vi "Test inner FIFO success.vi"() -> ()   [LabVIEW 2015]
uses:
  <vilib>/visionFPGA/Controls/IMAQ FPGA Image Size.ctl
  <vilib>/Platform/TimedLoop/XDataNode/timing_clust.ctl
  <vilib>/Platform/TimedLoop/XDataNode/nitl_modes.ctl
  <vilib>/Platform/TimedLoop/XDataNode/wakeup.ctl
  <vilib>/rvi/Emulation/niFpgaSctlEmulationGetInTimedLoop.vi
  <vilib>/rvi/Emulation/niFpgaEmulationReportErrorSimple.vi
  <vilib>/rvi/Emulation/niFpgaGetClockAttributes.vi
  <vilib>/rvi/Emulation/niFpgaCriticalErrorInLSC.vi
  <vilib>/rvi/DataTransferAndStorage/Container/Common/niFpgaContainerGetUniqueNameForEmu.vi
  <vilib>/rvi/DataTransferAndStorage/Container/Common/niFpgaContainerSetEmuInfo.vi
  <vilib>/rvi/eio/common/nirviEmuReportErrorAndStop.vi
  <vilib>/visionFPGA/Basics/FIFO to Pixel Bus/IMAQ FPGA FIFO to Pixel Bus RGB32x1.vi
  <vilib>/visionFPGA/Basics/Pixel Bus to FIFO/IMAQ FPGA Pixel Bus to FIFO U8x1.vi
  <vilib>/rvi/DataTransferAndStorage/Container/Common/niFpgaContainerExecOnDevCompGetState.vi
  <vilib>/rvi/Emulation/niFpgaEmulationIsFPGAContextNoSignature.vi
  <vilib>/rvi/errors/niFpgaSetErrorForExecOnDevCompSimple.vi
  <vilib>/rvi/FIFO/Fifo_Resource/nirvififoEmulationSetSize.vi
  <vilib>/rvi/FIFO/Fifo_Resource/nirviFifoEmulationQueueMgr.vi
  <instcachedir>/0/nirviFifoEmulationQueueMgr_E5CAEC123FF24DC58D834DCA3CDAA9B5.lvgen/nirviFifoEmulationQueueMgr_E5CAEC123FF24DC58D834DCA3CDAA9B5_001.vi
  <vilib>/rvi/FIFO/Fifo_Resource/nirvififoEmulationDetermineInputValidOut.vi
  <vilib>/rvi/FIFO/Fifo_Resource/nirvififoEmulationCreateLock.vi
  <vilib>/rvi/Emulation/niFpgaProcessEmulError.vi
  <vilib>/rvi/FIFO/Fifo_Resource/nirvififoEmulationObtainLock.vi
  <vilib>/rvi/FIFO/Fifo_Resource/nirvififoEmulationReleaseLock.vi
  <vilib>/rvi/occurrence/nirviWaitOnOccurrenceBase.vi
  <vilib>/rvi/errors/nirviReportUnexpectedCaseInternalError.vi
  <vilib>/rvi/errors/nirviReportUnexpectedCaseInternalError (U32).vi
  <vilib>/Utility/error.llb/Clear Errors.vi
  <vilib>/rvi/interface/RandomDataEmulation/niFpgaRandomDataHandleErrors.vi
  <vilib>/Platform/TimedLoop/XDataNode/XDataNode.xnode
  <vilib>/rvi/LocalResourceManager/LocalResourceManager.xnode
  <vilib>/rvi/DataTransferAndStorage/Container/XNode/niFpgaContainer.xnode
  <vilib>/rvi/FIFO/Fifo_Resource/niFpgaFifoEmulationRefIn.vi
  <vilib>/visionFPGA/NI_VDM_FPGA_Basics.lvlib
  <vilib>/Platform/TimedLoop/XDataNode/XDNodeRunTimeDep.lvlib
panel:
  out "appended array 2":u8[](array[numeric])
  out "appended array":i16[](array[numeric])
  out "Element":i16
  out "Output Valid":bool
  out "Pixel Data":u8
  out "Line count":i16
  in  "Image Size":T1={"Width"=640, "Height"=480}
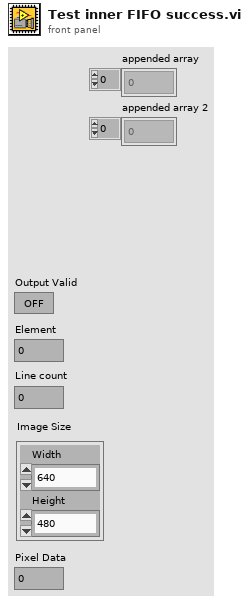
[diagram p1: front panel]
types:
  T1 = typedef "IMAQ FPGA Image Size.ctl" = cluster{"Width":u32, "Height":u32}
  T2 = typedef "XDNodeRunTimeDep.lvlib/timing_clust.ctl" = cluster{"Expected End [f-1]":u64, "Actual End [f-1]":u64, "Finished Late? [f-1]":bool, "Expected End [i-1]":u64, "Actual End [i-1]":u64, "Finished Late? [i-1]":bool, "Expected Start [i]":u64, "Actual Start [i]":u64, "Expected Start [f]":u64, "Actual Start [f]":u64, "Source Name":string, "Structure Name":string, "Period":i64, "Deadline":i64, "Offset":i64, "Start":i64, "Priority":i32, "Timeout":i32, "Mode":T3, "Wakeup Reason":T4, "Error":errorcluster, "Source Type":string, "Secondary Source Type":string, "Global End Time":u64, "Global Start Time":u64, "Frame Duration":u64, "Iteration Duration":u64, "Assigned CPU":i32, "I/O Scan Engine Mode":u32}
  T3 = typedef "XDNodeRunTimeDep.lvlib/nitl_modes.ctl" = enum32{"No Change", "Process missed periods, maintain original phase", "Discard missed periods, maintain original phase", "Process missed periods, ignore original phase", "Discard missed periods, ignore original phase"}
  T4 = typedef "XDNodeRunTimeDep.lvlib/wakeup.ctl" = enum32{"Normal", "Aborted", "Asynchronous wakeup", "Timing source error", "Timed loop error", "Timeout"}
  T5 = typedef "IMAQ FPGA Pixel Bus RGB32x1.ctl" = cluster{"Pixel Data":cluster{"A":u8, "R/H":u8, "G/S":u8, "B/L":u8}, "DV":bool, "EOL":bool, "EOI":bool, "Data Type":enum16{"RGB32 x 1"}}
  T6 = typedef "IMAQ FPGA Pixel Bus u8x1.ctl" = cluster{"Pixel Data":u8, "DV":bool, "EOL":bool, "EOI":bool, "Data Type":enum16{"U8 x 1"}}
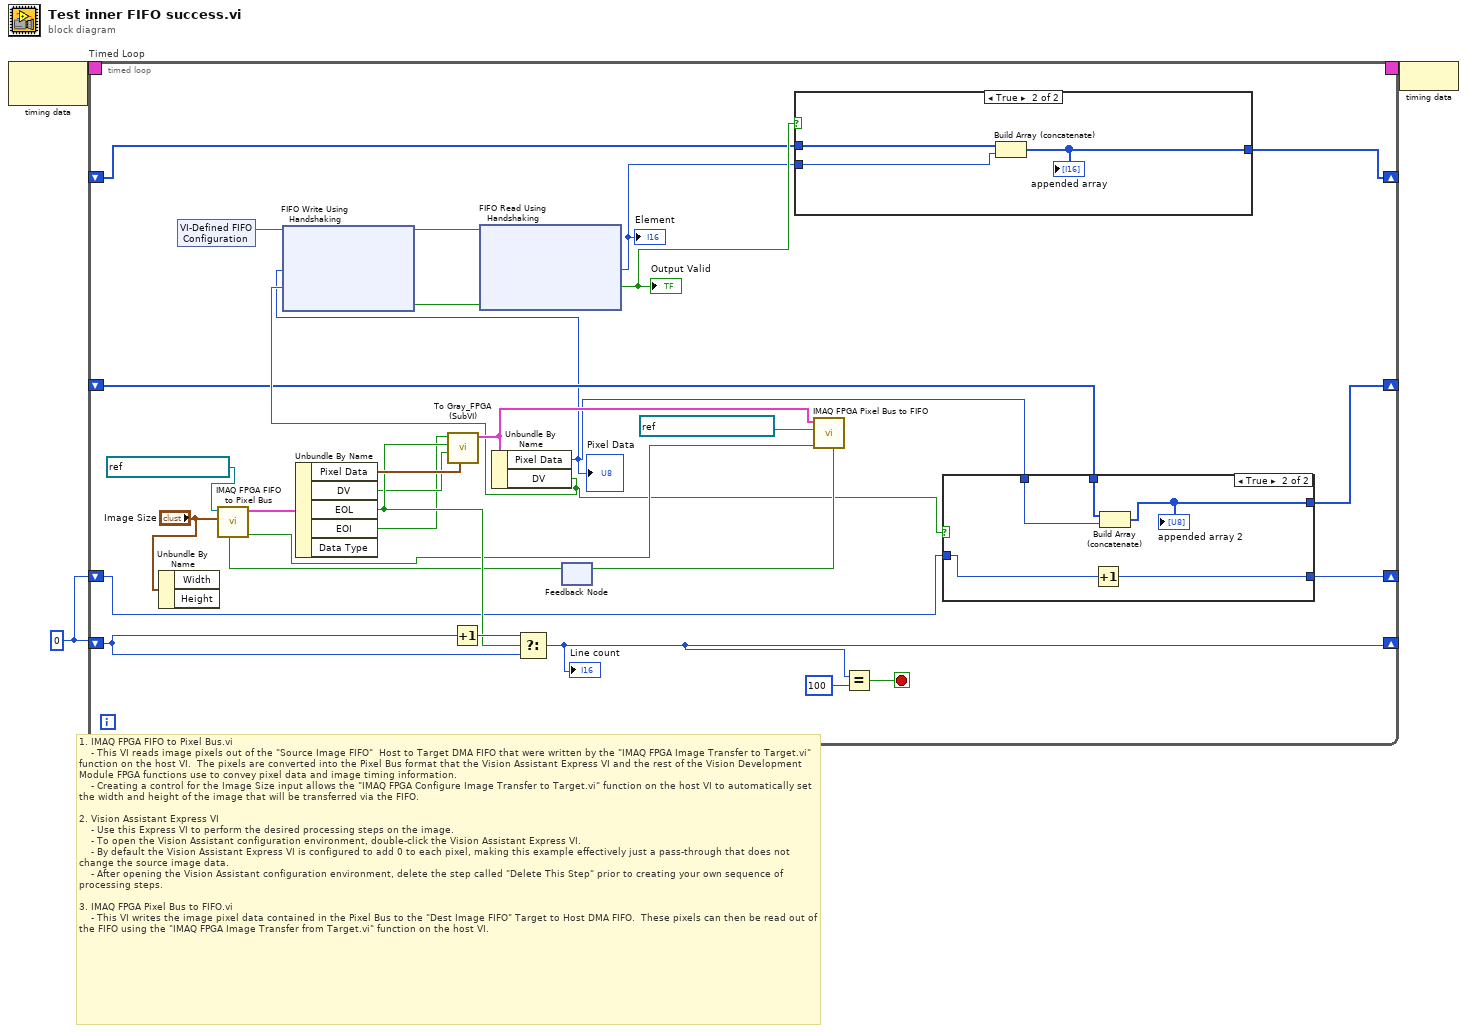
[diagram p0: block diagram]
diagram:
  w1 = i16 0
  # "1. IMAQ FPGA FIFO to Pixel Bus.vi\n    - This VI reads image pixels out of the \"Source Image FIFO\"  Host to Target DMA FIFO that were written by the \"IMAQ FPGA Image Transfer to Target.vi\" function on the host VI.  The pixels are converted into the Pixel Bus format that the Vision Assistant Express VI and the rest of the Vision Development Module FPGA functions use to convey pixel data and image timing information.\n    - Creating a control for the Image Size input allows the \"IMAQ FPGA Configure Image Transfer to Target.vi\" function on the host VI to automatically set the width and height of the image that will be transferred via the FIFO.\n\n2. Vision Assistant Express VI\n    - Use this Express VI to perform the desired processing steps on the image.\n    - To open the Vision Assistant configuration environment, double-click the Vision Assistant Express VI.\n    - By default the Vision Assistant Express VI is configured to add 0 to each pixel, making this example effectively just a pass-through that does not change the source image data.\n    - After opening the Vision Assistant configuration environment, delete the step called \"Delete This Step\" prior to creating your own sequence of processing steps.\n\n3. IMAQ FPGA Pixel Bus to FIFO.vi\n    - This VI writes the image pixel data contained in the Pixel Bus to the \"Dest Image FIFO\" Target to Host DMA FIFO.  These pixels can then be read out of the FIFO using the \"IMAQ FPGA Image Transfer from Target.vi\" function on the host VI."
  n1 = node-c288() -> (w3:T2)  [unwired: 1 in]
  n2 = timed-loop "Timed Loop" {
    timing: w3 -> [_]
    timing-out: [_] -> w2
    shift-right: [w12] -> _
    shift-left: w1 -> [w28]
    shift-right: [w15] -> _
    shift-left: w1 -> [w16]
    shift-right: [w8] -> _
    shift-left: _ -> [w7]
    shift-right: [w4] -> _
    shift-left: _ -> [w6]
    stop <- w13 stop-if-true
    n3 = Unbundle By Name("Image Size") -> ()  [unwired: 2 out]
    n4 = xnode "VI-Defined FIFO Configuration"() -> ("FIFO Out"=w20:refnum<k21>)
    n5 = Increment(x=w28) -> (x+1=w29:i16)
    n6 = feedback #1() -> (w21:bool)  [unwired: 1 in]
    n7 = call-poly <vilib>:"IMAQ FPGA FIFO to Pixel Bus.vi"("Ready For Output"=w21, "Image Size"="Image Size", "Source Image FIFO"=refnum<k21> "32it Source FIFO") -> ("Output Valid"=w23:bool, "Pixel Bus Out"=w31:T5)  [unwired: 6 in, 1 out]
    n8 = Unbundle By Name(w31) -> ("Pixel Data"=w27:cluster{"A":u8, "R/H":u8, "G/S":u8, "B/L":u8}, "DV"=w25:bool, "EOL"=w26:bool, "EOI"=w17:bool)  [unwired: 1 out]
    n9 = call "To Gray_FPGA (SubVI).vi"("Pixel Data"=w27, "DV"=w25, "EOL"=w26, "EOI"=w17) -> ("Pixel Bus In"=w24:T6)  [unwired: 7 in]
    n10 = Unbundle By Name(w24) -> ("Pixel Data"=w5:u8, "DV"=w14:bool)
    "Pixel Data" <- w5
    n11 = xnode ("FIFO Write Using Handshaking")("Element"=w5, "Input Valid"=w14, "FIFO In"=w20) -> ("Ready for Input"=w18:bool, "FIFO Out"=w19:refnum<k21>)
    n12 = xnode ("FIFO Read Using Handshaking")("Ready for Output"=w18, "FIFO In"=w19) -> ("Element"=w9:i16, "Output Valid"=w10:bool)  [unwired: 1 out]
    "Output Valid" <- w10
    "Element" <- w9
    n13 = Select(t=w29, s=w26, f=w28) -> (s? t:f=w12:i16)
    "Line count" <- w12
    n14 = case shown="True" w10 {
      tunnel: w9 -> [_ w37]
      tunnel: [w34 w36] -> w8
      tunnel: w7 -> [w34 w35]
      frame False {
      }
      frame True {
        n15 = Build Array (concatenate)(w35, w37) -> (w36:i16[])
        "appended array" <- w36
      }
    }
    n16 = call-poly <vilib>:"IMAQ FPGA Pixel Bus to FIFO.vi"("Input Valid"=w23, "Destination Image FIFO"=refnum<k21> "Dest 8bit FIFO Out", "Pixel Bus In"=w24) -> ("Ready for Input"=w22:bool)  [unwired: 8 in]
    n17 = feedback-in #1(w22) -> ()
    n18 = Equal?(x=w12, y=i16 100) -> (x = y?=w13:bool)
    n19 = case shown="True" w14 {
      tunnel: w16 -> [w39 w44]
      tunnel: [w39 w43] -> w15
      tunnel: w6 -> [w38 w42]
      tunnel: w5 -> [_ w41]
      tunnel: [w38 w40] -> w4
      frame False {
      }
      frame True {
        n20 = Increment(x=w44) -> (x+1=w43:i16)
        n21 = Build Array (concatenate)(w42, w41) -> (w40:u8[])
        "appended array 2" <- w40
      }
    }
  }
  n22 = node-c288(w2) -> ()
